vi "加载默认参数.vi"(11 "error IO":errorcluster) -> ()   [LabVIEW 2016, in "环境动力监测库.lvlib"]
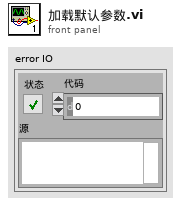
[diagram p1: front panel]
types:
  T1 = cluster{"功能启用":bool, "排气扇开启温度":dbl, "排气扇关闭温度":dbl}
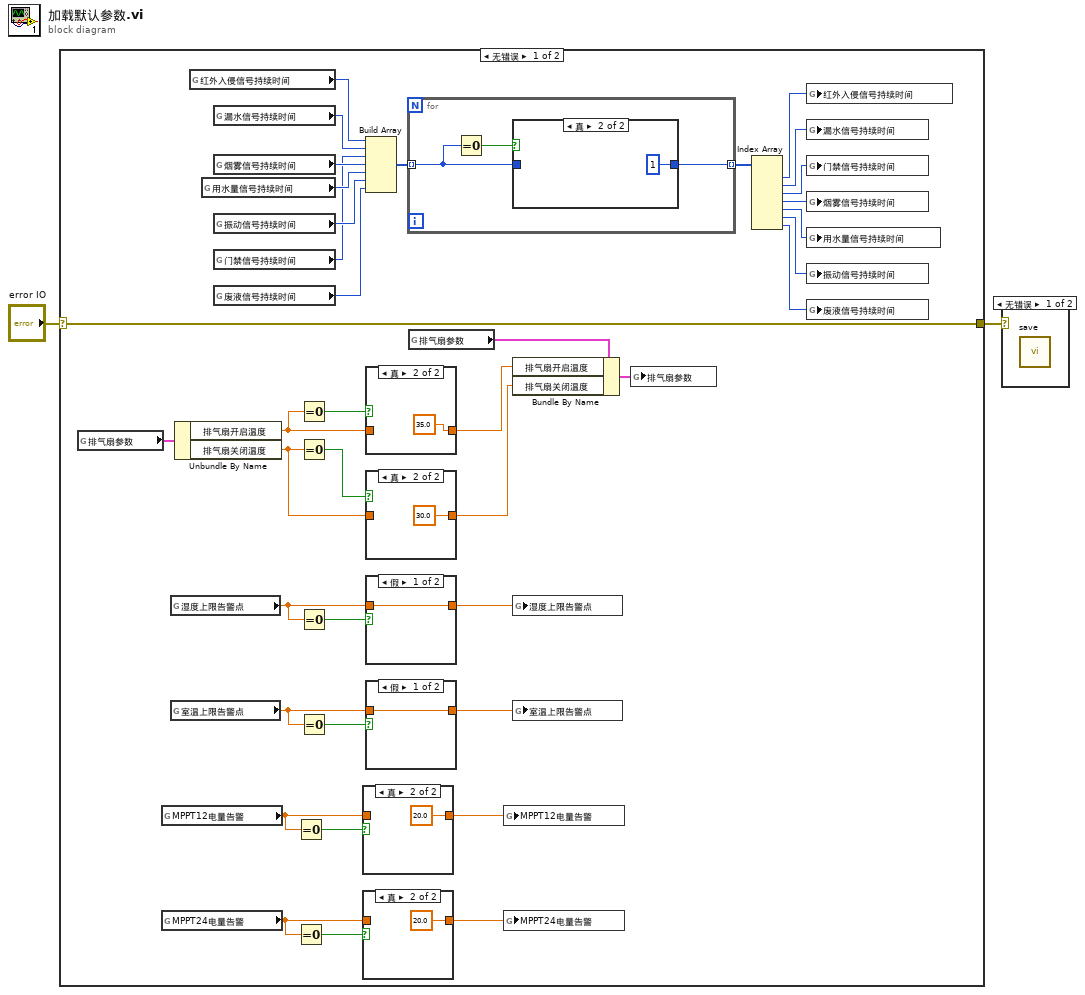
[diagram p0: block diagram]
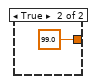
[diagram p6: hidden frame]
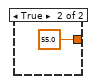
[diagram p7: hidden frame]
diagram:
  n1 = case shown="无错误" "error IO" {
    selector: "error IO" -> [w31 w58]
    tunnel: [w31 w58] -> w2
    frame No Error {
      n2 = global read "断电保存全局变量.vi" "排气扇参数"() -> (w40:T1)
      n3 = global read "断电保存全局变量.vi" "MPPT12电量告警"() -> (w8:dbl)
      n4 = global read "断电保存全局变量.vi" "MPPT24电量告警"() -> (w7:dbl)
      n5 = global read "断电保存全局变量.vi" "湿度上限告警点"() -> (w25:dbl)
      n6 = global read "断电保存全局变量.vi" "室温上限告警点"() -> (w26:dbl)
      n7 = Unbundle By Name(w40) -> ("排气扇开启温度"=w34:dbl, "排气扇关闭温度"=w32:dbl)
      n8 = global read "断电保存全局变量.vi" "红外入侵信号持续时间"() -> (w9:u32)
      n9 = global read "断电保存全局变量.vi" "用水量信号持续时间"() -> (w13:u32)
      n10 = global read "断电保存全局变量.vi" "漏水信号持续时间"() -> (w10:u32)
      n11 = global read "断电保存全局变量.vi" "烟雾信号持续时间"() -> (w12:u32)
      n12 = global read "断电保存全局变量.vi" "振动信号持续时间"() -> (w14:u32)
      n13 = global read "断电保存全局变量.vi" "门禁信号持续时间"() -> (w11:u32)
      n14 = global read "断电保存全局变量.vi" "废液信号持续时间"() -> (w15:u32)
      n15 = Equal To 0?(x=w8) -> (x = 0?=w6:bool)
      n16 = Equal To 0?(x=w7) -> (x = 0?=w5:bool)
      n17 = Equal To 0?(x=w34) -> (x = 0?=w35:bool)
      n18 = Equal To 0?(x=w32) -> (x = 0?=w33:bool)
      n19 = Equal To 0?(x=w25) -> (x = 0?=w27:bool)
      n20 = Equal To 0?(x=w26) -> (x = 0?=w28:bool)
      n21 = case shown="真" w6 {
        tunnel: [w41 20.0 ("室温上限告警点")] -> w3
        tunnel: w8 -> [w41 _]
        frame False {
        }
        frame True {
        }
      }
      n22 = case shown="真" w5 {
        tunnel: [w43 20.0 ("室温上限告警点")] -> w4
        tunnel: w7 -> [w43 _]
        frame False {
        }
        frame True {
        }
      }
      n23 = Build Array(w9, w10, w11, w12, w13, w14, w15) -> (w16:u32[])
      n24 = case shown="真" w35 {
        tunnel: [w56 35.0 ("值(信号)")] -> w37
        tunnel: w34 -> [w56 _]
        frame False {
        }
        frame True {
        }
      }
      n25 = case shown="真" w33 {
        tunnel: [w54 30.0 ("排气扇开启温度")] -> w36
        tunnel: w32 -> [w54 _]
        frame False {
        }
        frame True {
        }
      }
      n26 = case shown="假" w27 {
        tunnel: [w50 99.0 ("室温上限告警点")] -> w30
        tunnel: w25 -> [w50 _]
        frame False {
        }
        frame True {
        }
      }
      n27 = case shown="假" w28 {
        tunnel: [w52 55.0 ("室温上限告警点")] -> w29
        tunnel: w26 -> [w52 _]
        frame False {
        }
        frame True {
        }
      }
      n28 = for {
        tunnel: w16 -> [w45] mode=indexing
        tunnel: [w46] -> w17 mode=indexing
        n29 = Equal To 0?(x=w45) -> (x = 0?=w47:bool)
        n30 = case shown="真" w47 {
          tunnel: [w48 u32 1 ("红外入侵信号持续时间")] -> w46
          tunnel: w45 -> [w48 _]
          frame False {
          }
          frame True {
          }
        }
      }
      n31 = global read "断电保存全局变量.vi" "排气扇参数"() -> (w38:T1)
      n32 = global write "断电保存全局变量.vi" "MPPT12电量告警"(w3) -> ()
      n33 = global write "断电保存全局变量.vi" "MPPT24电量告警"(w4) -> ()
      n34 = Bundle By Name(cluster=w38, "排气扇开启温度"=w37, "排气扇关闭温度"=w36) -> (w39:T1)
      n35 = global write "断电保存全局变量.vi" "湿度上限告警点"(w30) -> ()
      n36 = global write "断电保存全局变量.vi" "室温上限告警点"(w29) -> ()
      n37 = global write "断电保存全局变量.vi" "排气扇参数"(w39) -> ()
      n38 = Index Array(array=w17) -> (element #1=w18:u32, element #2=w19:u32, element #3=w20:u32, element #4=w21:u32, element #5=w22:u32, element #6=w23:u32, element #7=w24:u32)  [unwired: 7 in]
      n39 = global write "断电保存全局变量.vi" "红外入侵信号持续时间"(w18) -> ()
      n40 = global write "断电保存全局变量.vi" "漏水信号持续时间"(w19) -> ()
      n41 = global write "断电保存全局变量.vi" "门禁信号持续时间"(w20) -> ()
      n42 = global write "断电保存全局变量.vi" "烟雾信号持续时间"(w21) -> ()
      n43 = global write "断电保存全局变量.vi" "用水量信号持续时间"(w22) -> ()
      n44 = global write "断电保存全局变量.vi" "振动信号持续时间"(w23) -> ()
      n45 = global write "断电保存全局变量.vi" "废液信号持续时间"(w24) -> ()
    }
    frame Error {
    }
  }
  n46 = case shown="无错误" w2 {
    frame No Error {
      n47 = call "save.vi"() -> ()  [unwired: 11 in, 1 out]
    }
    frame Error {
    }
  }
